vi "vERROR_All.vi"(8 "error in (no error)":errorcluster, 9 "結束時間":timestamp=timestamp(3738902301.8455286 s since 1904-01-01), 10 "開始時間":timestamp=timestamp(3738815886.436984 s since 1904-01-01), 11 "DBlink":string="Driver={ODBC Driver 17 for SQL Server};Server=localhost\\SQLEXPRESS;Database=ZDX201;UID=labview;PWD=Dsa@54137926") -> (0 "error out":errorcluster, 3 "故障Array":T1(array[cluster]))   [LabVIEW 2019]
uses:
  <vilib>/addons/database/Connection.llb/DB Tools Open Connec (String).vi
  <vilib>/addons/database/Connection.llb/Conn Execute.vi
  <vilib>/addons/database/Recordset.llb/Rec Fetch Recordset Data (R).vi
  <vilib>/addons/database/Recordset.llb/Rec Destroy - Connection.vi
  <vilib>/addons/database/_DB Variant To Data/Database Variant To Data.xnode
  <vilib>/addons/database/NI_Database_API.lvlib
panel:
  out "查詢結果":string="SELECT TOP (1000) [筆數]\n      ,[設備狀態]\n      ,[創建時間]\n  FROM [ZDX201].[dbo].[v_runcondition]\nwhere [創建時間] between '2022-06-23 15:58:06' AND '2022-06-24 15:58:21'"
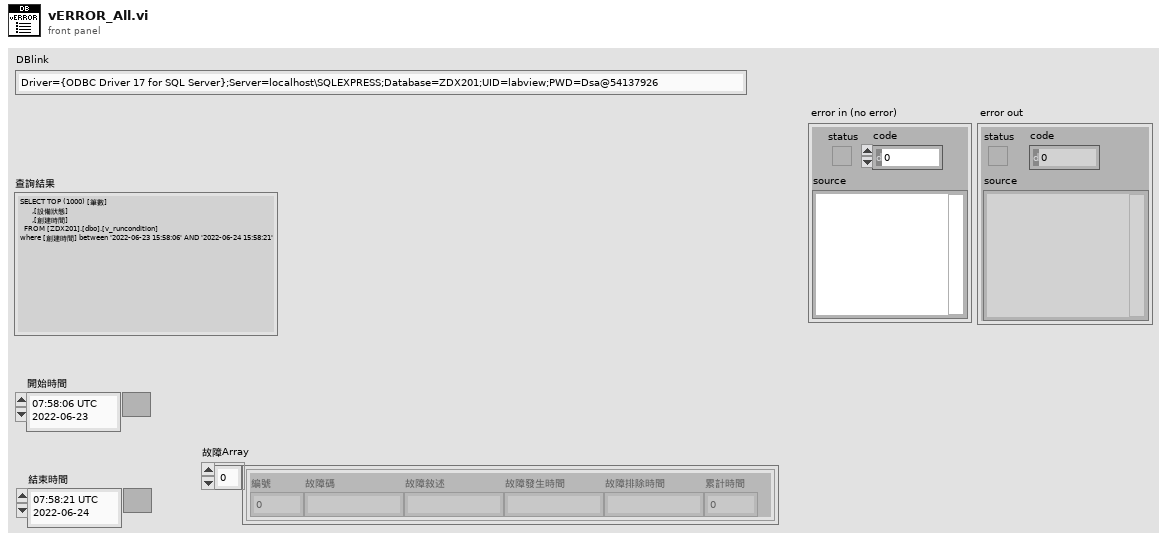
[diagram p1: front panel]
types:
  T1 = cluster{"編號":i16, "故障碼":string, "故障敘述":string, "故障發生時間":string, "故障排除時間":string, "累計時間":i16}[]
  T2 = typedef "NI_Database_API.lvlib/Conn ObjectReference.ctl" = refnum<k1>
  T3 = typedef "NI_Database_API.lvlib/Rec ObjectReference.ctl" = refnum<k1>
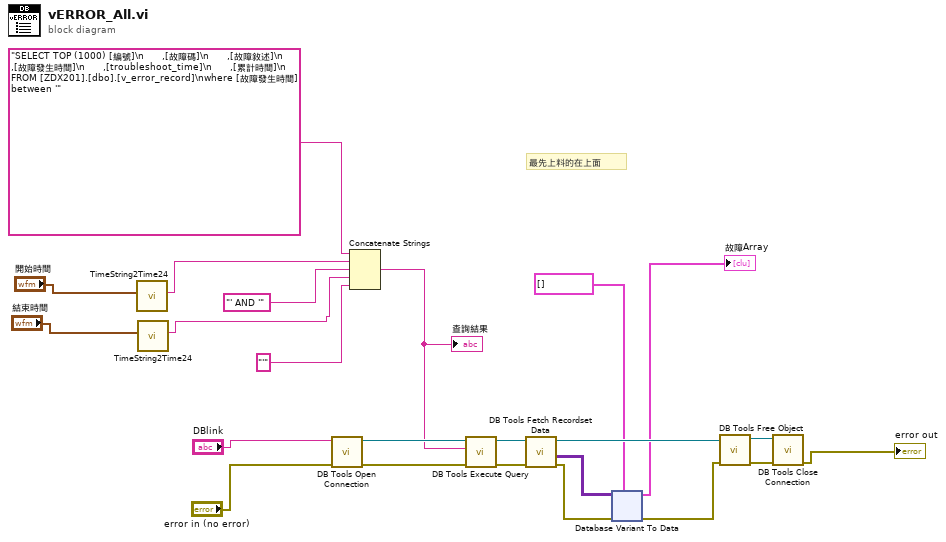
[diagram p0: block diagram]
diagram:
  # "最先上料的在上面"
  n1 = call "TimeString2Time24.vi"("Time Stamp"="開始時間") -> ("時間字串"=w2:string)  [unwired: 9 in, 1 out]
  n2 = call "TimeString2Time24.vi"("Time Stamp"="結束時間") -> ("時間字串"=w1:string)  [unwired: 9 in, 1 out]
  n3 = call-poly <vilib>:"DB Tools Open Connection.vi"("error in (no error)"="error in (no error)", "connection information"="DBlink") -> ("error out"=w23:errorcluster, "connection reference"=w22:T2)  [unwired: 6 in]
  n4 = Concatenate Strings("SELECT TOP (1000) [編號]\n      ,[故障碼]\n      ,[故障敘述]\n      ,[故障發生時間]\n      ,[troubleshoot_time]\n      ,[累計時間]\n  FROM [ZDX201].[dbo].[v_error_record]\nwhere [故障發生時間] between '", w2, "' AND '" ("string"), w1, "'" ("string")) -> (w5:string)
  "查詢結果" <- w5
  n5 = call-poly <vilib>:"DB Tools Execute Query.vi"("error in (no error)"=w23, "SQL query"=w5, "connection reference"=w22) -> ("error out"=w20:errorcluster, "recordset reference"=w21:T3)  [unwired: 5 in]
  n6 = call-poly <vilib>:"DB Tools Fetch Recordset Data.vi"("error in (no error)"=w20, "recordset reference"=w21) -> ("error out"=w15:errorcluster, "recordset data"=w14:variant[][], "recordset reference out"=w16:T3)  [unwired: 3 in]
  n7 = xnode "Database Variant To Data"("database variant"=w14, "error in (no error)"=w15, "type"=T1 [] ("Workplace")) -> ("data"=→"故障Array":T1, "error out"=w17:errorcluster)
  n8 = call-poly <vilib>:"DB Tools Free Object.vi"("error in (no error)"=w17, "recordset reference"=w16) -> ("error out"=w18:errorcluster, "connection reference"=w19:T2)  [unwired: 8 in]
  n9 = call <vilib>:"DB Tools Close Connection.vi"("error in (no error)"=w18, "connection reference"=w19) -> ("error out"=→"error out":errorcluster)  [unwired: 5 in]
